vi "Read BBM Fiducials.vi"(8 "error in":errorcluster, 9 "Slot":u32, 10 "Chuck":u32, 11 "CameraTool in":refnum<class "CameraTool Class.lvclass">) -> (0 "error out":errorcluster, 3 "CameraTool out":refnum<class "CameraTool Class.lvclass">)   [LabVIEW 2011, in "CameraTool Class.lvclass"]
uses:
  CameraTool Class.lvclass
  WorkTable Class/WorkTable Class.lvclass
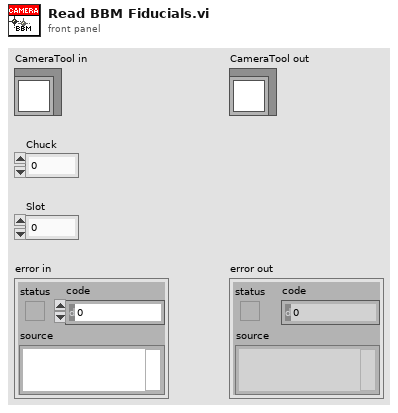
[diagram p1: front panel]
types:
  T1 = cluster{"Fiducial Type":string, "Selection Criteria":enum16{"Single", "Top", "Bottom"}}
  T2 = typedef "Worktable_BBM Slot.ctl" = cluster{"BBM Slot State":enum16{"Empty", "Unglued", "Stamped", "PartOnTop", "Weighted", "Unpotted", "Potted"}, "BBM Type":enum16{"BBM", "GlassSlide"}, "HDI Type":enum16{"HDI", "Polyimide"}, "Vacuum Channel":u8, "Location/Orientation BBM":T3, "Location/Orientation HDI":T3}
  T3 = typedef "Position_Orientation.ctl" = cluster{"Center":refnum<class "Vec3d Class.lvclass">, "Orientation":refnum<class "Orient3d Class.lvclass">}
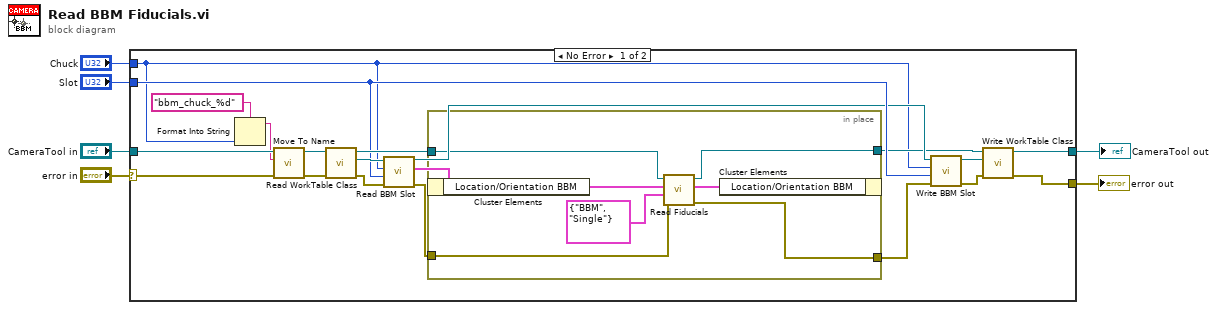
[diagram p0: block diagram]
diagram:
  n1 = case shown="No Error" "error in" {
    selector: "error in" -> [w20 w35]
    tunnel: [w21 w35] -> w4
    tunnel: "CameraTool in" -> [w22 w34]
    tunnel: "Chuck" -> [w8 _]
    tunnel: "Slot" -> [w16 _]
    tunnel: [w15 w34] -> w1
    frame No Error {
      n2 = Format Into String(format string="bbm_chuck_%d", w8) -> (resulting string=w7:string)  [unwired: 2 in, 1 out]
      n3 = call-dynamic "Move To Name.vi"("error in"=w20, "Destination Name"=w7, "Gantry in"=w22) -> ("error out"=w26:errorcluster, "Gantry out"=w25:refnum<class "CameraTool Class.lvclass">)  [unwired: 7 in]
      n4 = call-dynamic "Read WorkTable Class.vi"("error in"=w26, "Gantry Class in"=w25) -> ("error out"=w23:errorcluster, "WorkTable Class.lvclass"=w24:refnum<class "WorkTable Class.lvclass">, "Gantry Class out"=w18:refnum<class "CameraTool Class.lvclass">)  [unwired: 7 in]
      n5 = call-dynamic "Read BBM Slot.vi"("error in (no error)"=w23, "Slot Number"=w16, "Chuck Number"=w8, "WorkTable Class in"=w24) -> ("error out"=w19:errorcluster, "BBM Slot"=w17:T2, "WorkTable Class out"=w12:refnum<class "WorkTable Class.lvclass">)  [unwired: 5 in]
      n6 = in-place {
        in-place-border: w19 -> [w31]
        in-place-border: w18 -> [w29]
        in-place-border: [w30] -> w11
        in-place-border: [w28] -> w10
        n7 = in-place-cluster #1(w17) -> ("Location/Orientation BBM"=w33:T3)
        n8 = call-dynamic "Read Fiducials.vi"("error in"=w31, "Fiducial Acquisition Parameters"=T1 {"Fiducial Type"="BBM", "Selection Criteria"=enum."Single"}, "Location/Orientation in"=w33, "CameraTool in"=w29) -> ("error out"=w30:errorcluster, "Location/Orientation out"=w32:T3, "CameraTool out"=w28:refnum<class "CameraTool Class.lvclass">)  [unwired: 5 in]
        n9 = in-place-cluster #1("Location/Orientation BBM"=w32) -> ()  [unwired: 1 out]
      }
      n10 = call-dynamic "Write BBM Slot.vi"("error in (no error)"=w11, "Slot Number"=w16, "Chuck Number"=w8, "WorkTable Class in"=w12) -> ("error out"=w13:errorcluster, "WorkTable Class out"=w14:refnum<class "WorkTable Class.lvclass">)  [unwired: 6 in]
      n11 = call-dynamic "Write WorkTable Class.vi"("error in (no error)"=w13, "WorkTable Class.lvclass"=w14, "Gantry Class in"=w10) -> ("error out"=w21:errorcluster, "Gantry Class out"=w15:refnum<class "CameraTool Class.lvclass">)  [unwired: 7 in]
    }
    frame Error {
    }
  }
  "CameraTool out" <- w1
  "error out" <- w4
